vi "CANOpen EDS value to block.vi"(10 "DataType":T1 items=[""=0, "BOOLEAN"=1, "INTEGER8"=2, "INTEGER16"=3, "INTEGER32"=4, "UNSIGNED8"=5, "UNSIGNED16"=6, "UNSIGNED32"=7, "REAL32"=8, "VISIBLE_STRING"=9, "OCTET_STRING"=10, "UNICODE_STRING"=11, "TIME_OF_DAY"=12, "TIME_DIFFERENCE"=13, "DOMAIN"=15, "INTEGER24"=16, "REAL64"=17, "INTEGER40"=18, "INTEGER48"=19, "INTEGER56"=20, "INTEGER64"=21, "UNSIGNED24"=22, "UNSIGNED40"=24, "UNSIGNED48"=25, "UNSIGNED56"=26, "UNSIGNED64"=27], 11 "Translated value":i64) -> (3 "Block Data":u8[](array[numeric]))   [LabVIEW 2013, in "CANOpen Addon Custom Device.lvlib"]
uses:
  CANOpen Addon Custom Device.lvlib
  EDS/control/Data Type.ctl
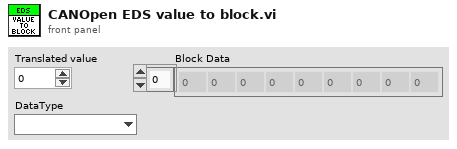
[diagram p1: front panel]
types:
  T1 = typedef "Data Type.ctl" = u16
  T2 = enum16{"big-endian, network order", "native, host order", "little-endian"}
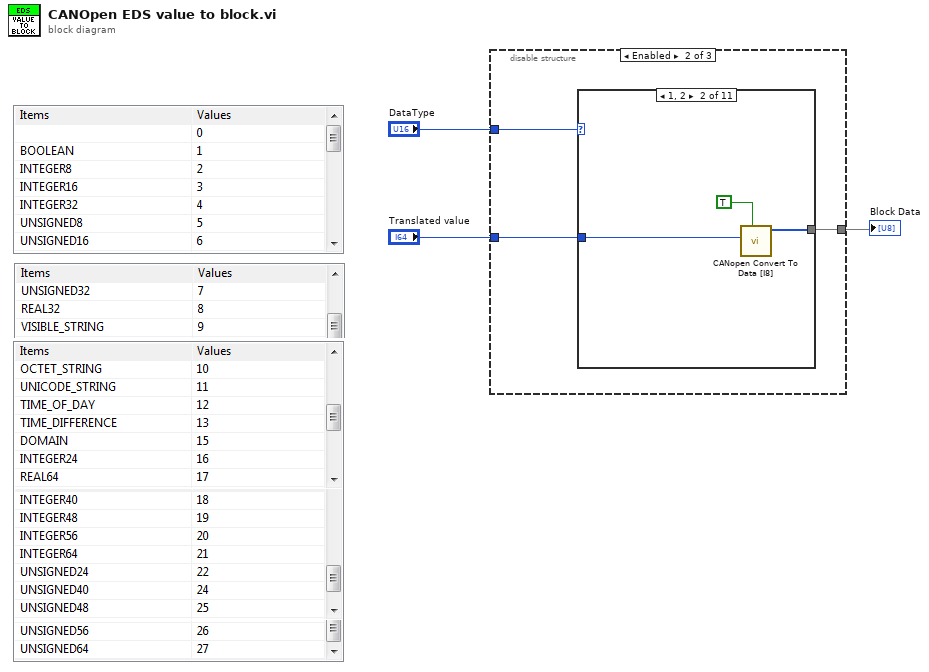
[diagram p0: block diagram]
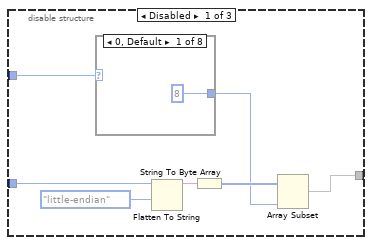
[diagram p2: hidden frame]
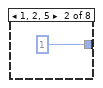
[diagram p3: hidden frame]
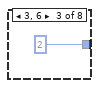
[diagram p4: hidden frame]
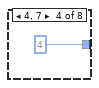
[diagram p5: hidden frame]
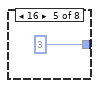
[diagram p6: hidden frame]
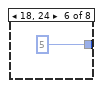
[diagram p7: hidden frame]
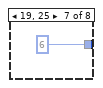
[diagram p8: hidden frame]
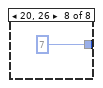
[diagram p9: hidden frame]
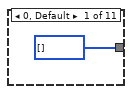
[diagram p10: hidden frame]
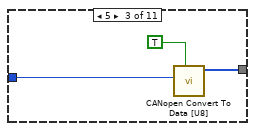
[diagram p11: hidden frame]
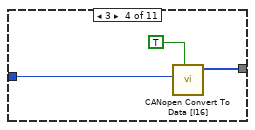
[diagram p12: hidden frame]
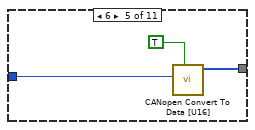
[diagram p13: hidden frame]
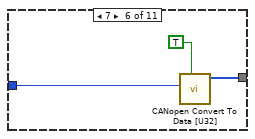
[diagram p14: hidden frame]
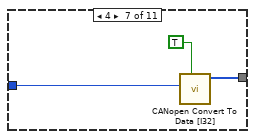
[diagram p15: hidden frame]
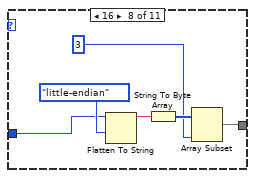
[diagram p16: hidden frame]
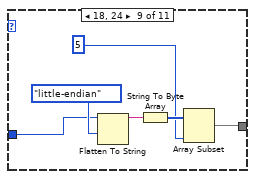
[diagram p17: hidden frame]
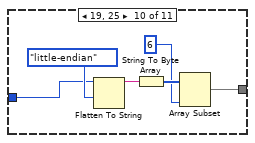
[diagram p18: hidden frame]
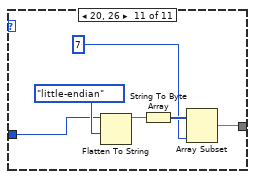
[diagram p19: hidden frame]
diagram:
  n1 = disable-structure shown="Enabled" {
    disable-tunnel: "DataType" -> [w7 w21 _]
    disable-tunnel: [w5 w20 _] -> w2
    disable-tunnel: "Translated value" -> [w4 w19 _]
    frame Disabled {
      n2 = case shown="0, Default" w7 {
        tunnel: [8 ("length") 1 ("length") 2 ("length") 4 ("length") 3 ("length") 5 ("length") 6 ("length") 7 ("length")] -> w6
        frame 0, Default {
        }
        frame 1, 2, 5 {
        }
        frame 3, 6 {
        }
        frame 4, 7 {
        }
        frame 16 {
        }
        frame 18, 24 {
        }
        frame 19, 25 {
        }
        frame 20, 26 {
        }
      }
      n3 = Flatten To String(anything=w4, byte order (0:big-endian, network order)=T2."little-endian") -> (data string=w9:string)  [unwired: 2 in, 2 out]
      n4 = String To Byte Array(string=w9) -> (unsigned byte array=w8:u8[])
      n5 = Array Subset(array=w8, length=w6) -> (w5:u8[])  [unwired: 1 in]
    }
    frame Enabled {
      n6 = case shown="1, 2" w21 {
        tunnel: [u8[] [] ("Block Data") w23 w27 w29 w33 w36 w40 w41 w49 w54 w61] -> w20
        tunnel: w19 -> [_ w24 w28 w30 w34 w35 w38 w43 w48 w55 w60]
        frame 0, Default {
        }
        frame 1, 2 {
          n7 = call <vilib>:"CANopen Convert To Data [I8].vi"("trim"=TRUE, "signed 8-bit integer"=w24) -> ("CANopen data out"=w23:u8[])  [unwired: 8 in, 1 out]
        }
        frame 5 {
          n8 = call <vilib>:"CANopen Convert To Data [U8].vi"("trim"=TRUE, "unsigned 8-bit integer"=w28) -> ("CANopen data out"=w27:u8[])  [unwired: 8 in, 1 out]
        }
        frame 3 {
          n9 = call <vilib>:"CANopen Convert To Data [I16].vi"("trim"=TRUE, "signed 16-bit integer"=w30) -> ("CANopen data out"=w29:u8[])  [unwired: 8 in, 1 out]
        }
        frame 6 {
          n10 = call <vilib>:"CANopen Convert To Data [U16].vi"("trim"=TRUE, "unsigned 16-bit integer"=w34) -> ("CANopen data out"=w33:u8[])  [unwired: 8 in, 1 out]
        }
        frame 7 {
          n11 = call <vilib>:"CANopen Convert To Data [U32].vi"("trim"=TRUE, "unsigned 32-bit integer"=w35) -> ("CANopen data out"=w36:u8[])  [unwired: 8 in, 1 out]
        }
        frame 4 {
          n12 = call <vilib>:"CANopen Convert To Data [I32].vi"("trim"=TRUE, "signed 32-bit integer"=w38) -> ("CANopen data out"=w40:u8[])  [unwired: 8 in, 1 out]
        }
        frame 16 {
          n13 = Flatten To String(anything=w43, byte order (0:big-endian, network order)=T2."little-endian") -> (data string=w45:string)  [unwired: 2 in, 2 out]
          n14 = String To Byte Array(string=w45) -> (unsigned byte array=w44:u8[])
          n15 = Array Subset(array=w44, length=3) -> (w41:u8[])  [unwired: 1 in]
        }
        frame 18, 24 {
          n16 = Flatten To String(anything=w48, byte order (0:big-endian, network order)=T2."little-endian") -> (data string=w51:string)  [unwired: 2 in, 2 out]
          n17 = String To Byte Array(string=w51) -> (unsigned byte array=w50:u8[])
          n18 = Array Subset(array=w50, length=5) -> (w49:u8[])  [unwired: 1 in]
        }
        frame 19, 25 {
          n19 = Flatten To String(anything=w55, byte order (0:big-endian, network order)=T2."little-endian") -> (data string=w57:string)  [unwired: 2 in, 2 out]
          n20 = String To Byte Array(string=w57) -> (unsigned byte array=w56:u8[])
          n21 = Array Subset(array=w56, length=6) -> (w54:u8[])  [unwired: 1 in]
        }
        frame 20, 26 {
          n22 = Flatten To String(anything=w60, byte order (0:big-endian, network order)=T2."little-endian") -> (data string=w63:string)  [unwired: 2 in, 2 out]
          n23 = String To Byte Array(string=w63) -> (unsigned byte array=w62:u8[])
          n24 = Array Subset(array=w62, length=7) -> (w61:u8[])  [unwired: 1 in]
        }
      }
    }
    frame Disabled {
    }
  }
  "Block Data" <- w2
